vi "OP60_Push_Pass_List.vi"(11 "Refnum in":T1) -> (0 "error out":errorcluster, 3 "Array":string[][](array[string]))   [LabVIEW 2020]
uses:
  <vilib>/addons/database/Connection.llb/Conn ObjectReference.ctl
  <vilib>/addons/database/Connection.llb/Conn Execute.vi
  <vilib>/addons/database/Recordset.llb/Rec Fetch Recordset Data (R).vi
  <vilib>/addons/database/Recordset.llb/Rec Destroy - Connection.vi
  <vilib>/addons/database/NI_Database_API.lvlib
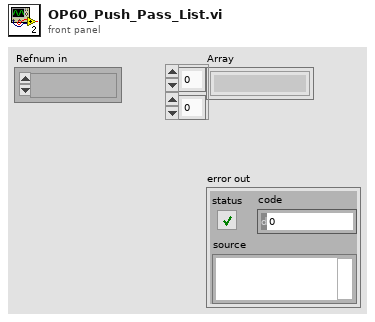
[diagram p1: front panel]
types:
  T1 = typedef "NI_Database_API.lvlib/Conn ObjectReference.ctl" = refnum<k1>
  T2 = typedef "NI_Database_API.lvlib/Rec ObjectReference.ctl" = refnum<k1>
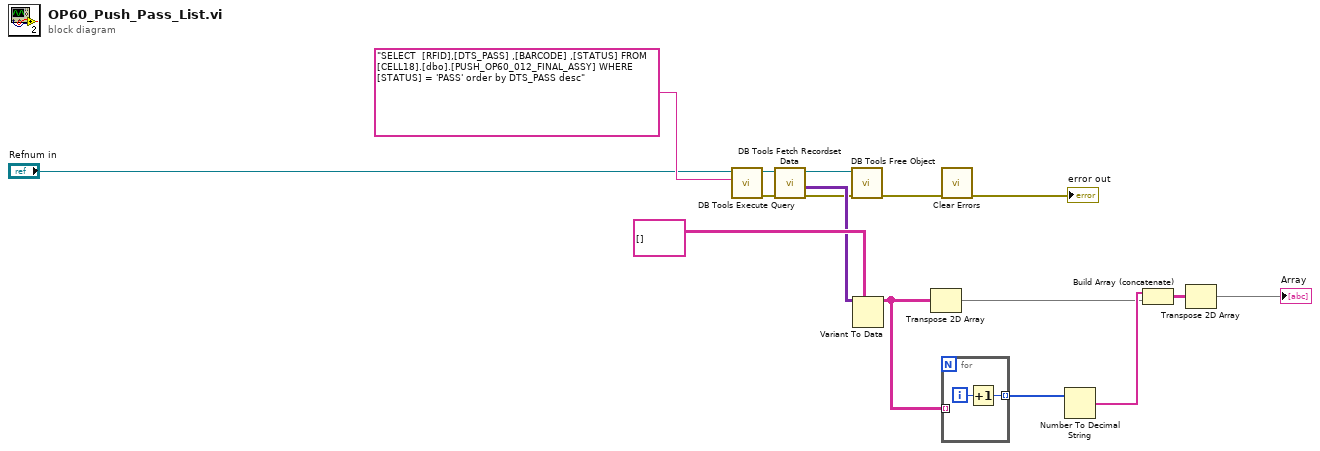
[diagram p0: block diagram]
diagram:
  n1 = call-poly <vilib>:"DB Tools Execute Query.vi"("SQL query"="SELECT  [RFID],[DTS_PASS] ,[BARCODE] ,[STATUS] FROM [CELL18].[dbo].[PUSH_OP60_012_FINAL_ASSY] WHERE [STATUS] = 'PASS' order by DTS_PASS desc" ("condition"), "connection reference"="Refnum in") -> ("error out"=w4:errorcluster, "recordset reference"=w3:T2)  [unwired: 6 in]
  n2 = call-poly <vilib>:"DB Tools Fetch Recordset Data.vi"("error in (no error)"=w4, "recordset reference"=w3) -> ("error out"=w5:errorcluster, "recordset data"=w8:variant[][], "recordset reference out"=w2:T2)  [unwired: 3 in]
  n3 = call-poly <vilib>:"DB Tools Free Object.vi"("error in (no error)"=w5, "recordset reference"=w2) -> ("error out"=w16:errorcluster)  [unwired: 8 in, 1 out]
  n4 = Variant To Data(type=string[][] [], Variant=w8) -> (data=w10:string[][])  [unwired: 1 in, 1 out]
  n5 = Transpose 2D Array(2D array=w10) -> (transposed array=w13:string[][])
  n6 = call <vilib>:"Clear Errors.vi"("error in (no error)"=w16) -> ("error out"=→"error out":errorcluster)  [unwired: 5 in, 1 out]
  n7 = for {
    tunnel: w10 -> [_] mode=indexing
    tunnel: [w17] -> w11 mode=indexing
    i -> [w18]
    n8 = Increment(x=w18) -> (x+1=w17:i32)
  }
  n9 = Number To Decimal String(number=w11) -> (decimal integer string=w14:string[])  [unwired: 1 in]
  n10 = Build Array (concatenate)(w14, w13) -> (w12:string[][])
  n11 = Transpose 2D Array(2D array=w12) -> (transposed array=→"Array":string[][])
